vi "Write_CamUserSync.vi"(10 "cam_USER_SYNC":i16) -> ()   [LabVIEW 2023, in "Cam Data.lvlib"]
uses:
  Cam Data.lvlib
panel:
  in  "Array":i32[](array[numeric])
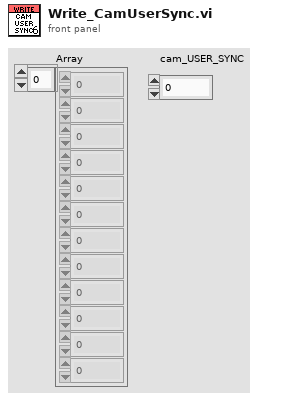
[diagram p1: front panel]
types:
  T1 = cluster{"Address IP":string, "Rack":i32, "Slot ":i32, "DB Number":i32, "Start":i32, "Amount":i32, "Word Length":i32}
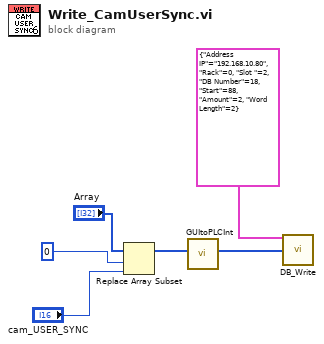
[diagram p0: block diagram]
diagram:
  n1 = Replace Array Subset(array="Array", new element="cam_USER_SYNC", index=0) -> (w2:i32[])
  n2 = call "GUItoPLCInt.vi"("Real Input Array"=w2) -> ("DB Output Array"=w6:u8[])  [unwired: 10 in]
  n3 = call "DB_Write.vi"("Input Params"=T1 {"Address IP"="192.168.10.80", "Rack"=0, "Slot "=2, "DB Number"=18, "Start"=88, "Amount"=2, "Word Length"=2}, "Array"=w6) -> ()  [unwired: 13 in, 1 out]
